vi "midiPlayer.announcements.get.vi"(11 "midi":refnum<class "midi.lvclass">) -> (2 "midiPlayer.Announcements":refnum<user-event>)   [LabVIEW 2020, in "midi.lvclass"]
uses:
  midi.lvclass
  midi.lvclass/midi.ctl
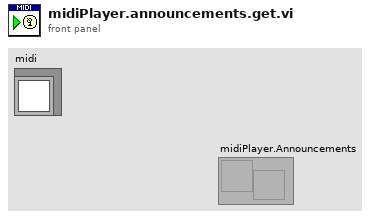
[diagram p1: front panel]
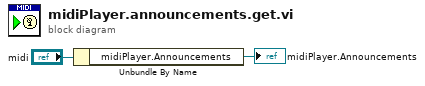
[diagram p0: block diagram]
diagram:
  n1 = Unbundle By Name("midi") -> ("midiPlayer.Announcements"=→"midiPlayer.Announcements":refnum<user-event>)
